vi "2014FullVi.vi"() -> ()   [LabVIEW 2014]
doc: "Use this template to build a standard state machine design pattern. Each state executes code and determines which state to transition to. Contrast this design pattern with the User Interface Event Handler pattern, in which code executes in response to user actions. Contrast this design pattern also with the Queued Message Handler pattern, in which each message handling code can queue zero or more new messages.\nNote: This template does not contain the most recent programming guidelines recommended by National Instruments. For a complete, project-based implementation of the Standard State Machine pattern, use the Create Project dialog box instead of this template."
uses:
  <vilib>/Math Plots/3D Math Plots/3D Bar/3D Bar Datatype/3D Bar Datatype.lvclass
  <vilib>/Math Plots/3D Math Plots/3D Bar/3D Bar Datatype/Public/Plot Helper (Vector).vi
  <vilib>/express/express arith-compare/Formula/XNode/ExpressFormulaBlockNode.xnode
  <vilib>/University of Leeds/Kinesthesia Toolkit for Microsoft Kinect/_Polymorphic Configure/Event-Depth, Skeleton and Video.vi
  <vilib>/University of Leeds/Kinesthesia Toolkit for Microsoft Kinect/_Polymorphic Read/Read-Depth, Skeleton and Video.vi
  <vilib>/Math Plots/3D Math Plots/3D Bar/3D Bar XCtrl/3D Bar.xctl
  Control 1.ctl
panel:
  in  "Which Joint? (2)":T1(ring)
  out "Joint Coordinates (2)":dbl[](array[numeric])
  out "Joint Coordinates (1)":dbl[](array[numeric])
  in  "Which Joint? (1)":T1(ring)
  out "Base DD":dbl[](array[numeric])
  out "Total DD":dbl[](array[numeric])
  in  "1/2 Twist":dbl[](array[numeric])
  in  "360 Somersault":T2
  in  "1/4 Rotation":dbl[](array[numeric])
  in  "Position":string[](array[combo])
  in  "Skill":string[](array[combo])
  in  "FIG Shorthand":string[](array[string])
  out "Average Jump Time":dbl format="%#.3g"
  out "Standard \nDeviation":dbl format="%#.4g"
  out "Tramp contact":bool
  out "?":refnum<class "3D Plot Datatype.lvclass">[](xcontrol)
  out "Total Air Time":dbl format="%#.3g"
  out "Number of Total Jumps":i32
  out "Number of Official Jumps":i32
  in  "Start Official Jumps":bool
  out "Final Jump Times":dbl[](array[numeric])
  out "Trampoline Time":dbl[](array[numeric])
  out "Air Time":dbl[](array[numeric])
  in  "Stop":bool
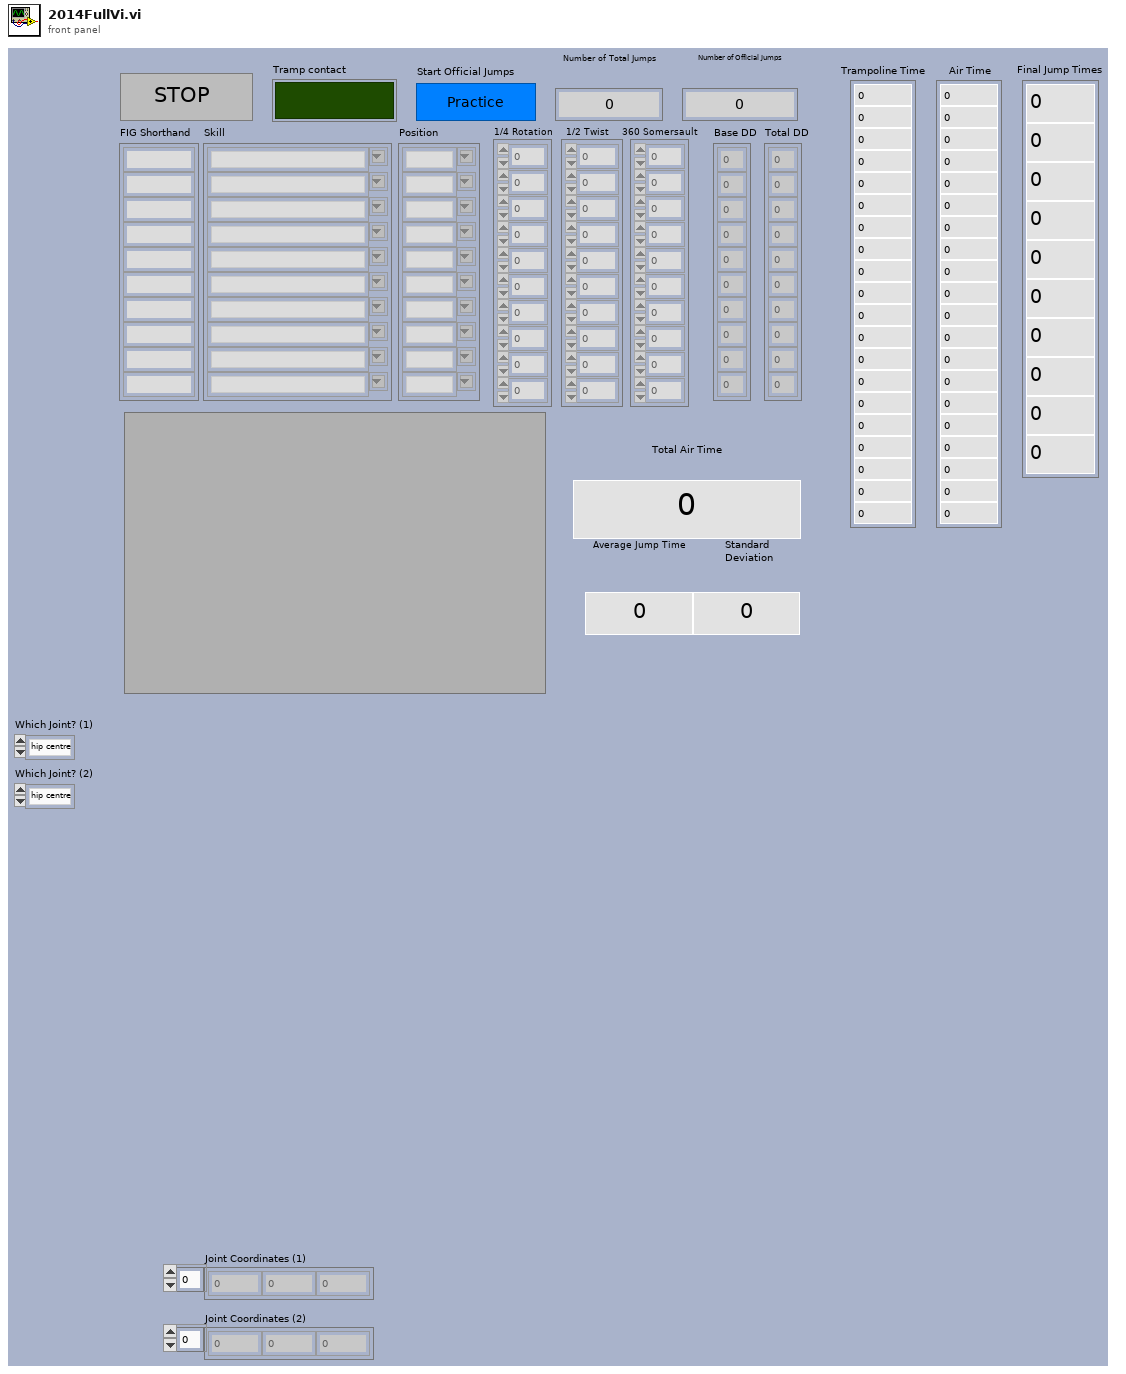
[diagram p1: front panel]
types:
  T1 = enum16{"hip centre", "spine", "shoulder centre", "head", "shoulder left", "elbow left", "wrist left", "hand left", "shoulder right", "elbow right", "wrist right", "hand right", "hip left", "knee left", "ankle left", "foot left", "hip right", "knee right", "ankle right", "foot right"}
  T2 = typedef "Control 1.ctl" = dbl[]
  T3 = cluster{"Start Time":dbl, "Air Time Array ":dbl[], "Tramp Time Array":dbl[], "Number of Jumps  ":i32, "Final Time Array":dbl[], "Number of Final Jumps":i32, "Tramp switch":bool}
  T4 = enum16{"Initialize", "acquire", "analyze", "display", "Stop"}
  T5 = cluster{cluster{"reference out":refnum<k24>, "KinectSensors":refnum<k24>}, "get_Item":refnum<k24>}
  T6 = cluster{"reference out":refnum<k24>, "KinectSensors":refnum<k24>, "SkeletonStream":refnum<k24>, "DepthStream":refnum<k24>, "ColorStream":refnum<k24>, refnum<k24>[], "get_Item":refnum<k24>}
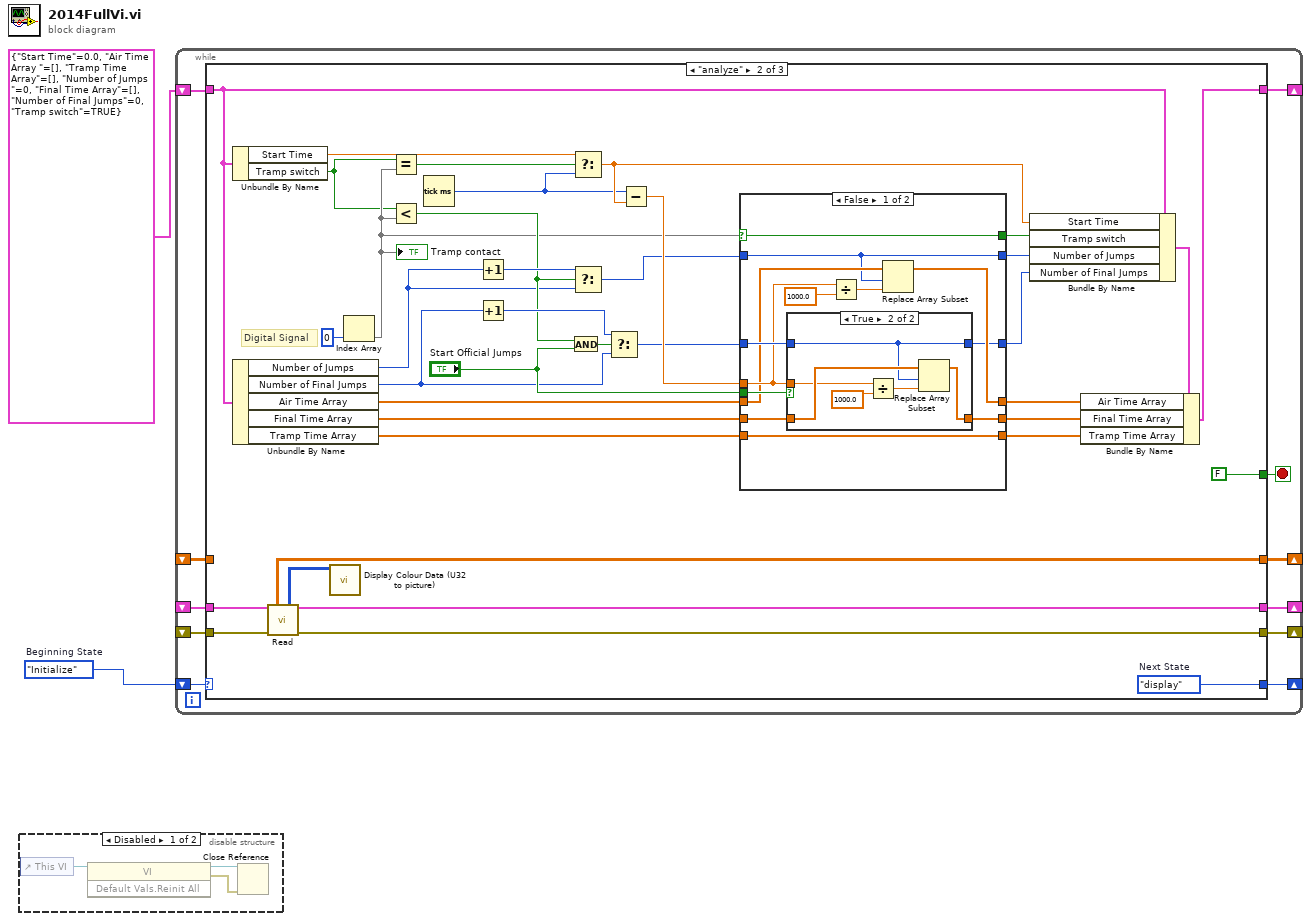
[diagram p0: block diagram]
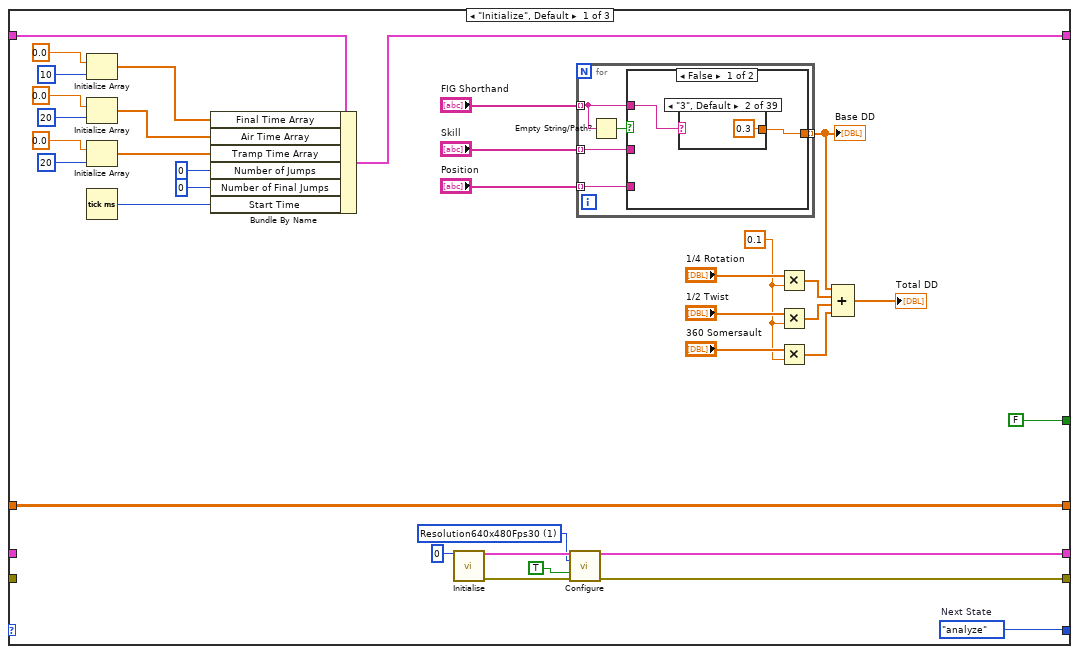
[diagram p3: hidden frame]
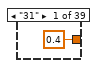
[diagram p4: hidden frame]
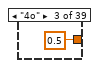
[diagram p5: hidden frame]
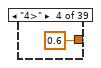
[diagram p6: hidden frame]
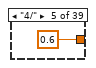
[diagram p7: hidden frame]
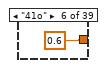
[diagram p8: hidden frame]
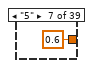
[diagram p9: hidden frame]
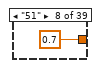
[diagram p10: hidden frame]
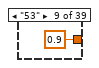
[diagram p11: hidden frame]
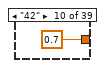
[diagram p12: hidden frame]
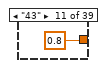
[diagram p13: hidden frame]
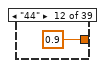
[diagram p14: hidden frame]
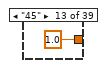
[diagram p15: hidden frame]
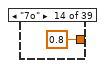
[diagram p16: hidden frame]
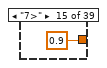
[diagram p17: hidden frame]
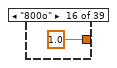
[diagram p18: hidden frame]
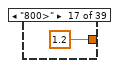
[diagram p19: hidden frame]
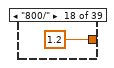
[diagram p20: hidden frame]
diagram:
  w2 = T4."Initialize"  # Beginning State
  n1 = disable-structure shown="Disabled" {
    frame Disabled {
      n2 = control-ref of="This VI"() -> (w5:refnum<vi>)
      n3 = invoke class="VI" method="Default Vals.Reinit All"(reference=w5) -> (reference out=w4:refnum<vi>, error out=w3:errorcluster)  [unwired: 2 in, 1 out]
      n4 = Close Reference(reference=w4, error in (no error)=w3) -> ()  [unwired: 1 out]
    }
    frame Enabled {
    }
  }
  n5 = while {
    shift-right: [w13] -> _
    shift-left: w2 -> [w16]
    shift-right: [w14] -> _
    shift-left: T3 {"Start Time"=0.0, "Air Time Array "=[], "Tramp Time Array"=[], "Number of Jumps  "=0, "Final Time Array"=[], "Number of Final Jumps"=0, "Tramp switch"=TRUE} -> [w15]
    shift-right: [w11] -> _
    shift-left: _ -> [w9]
    shift-right: [w10] -> _
    shift-left: _ -> [w8]
    shift-right: [w7] -> _
    shift-left: _ -> [w6]
    stop <- w12 stop-if-true
    n6 = case shown="\"analyze\"" w16 {
      tunnel: [w52 w224 w284] -> w13
      tunnel: w15 -> [w51 w209 w281]
      tunnel: [w43 w201 w281] -> w14
      tunnel: [FALSE FALSE w282] -> w12
      tunnel: [w19 w188 w256] -> w11
      tunnel: [w18 w189 w258] -> w10
      tunnel: w9 -> [_ w191 w256]
      tunnel: w8 -> [_ w190 w259]
      tunnel: [w17 w187 w257] -> w7
      tunnel: w6 -> [w17 _ w257]
      frame "Initialize", Default {
        w21 = 1 items=["Undefined", "Resolution640x480Fps30", "Resolution320x240Fps30", "Resolution80x60Fps30"] ("Depth Stream Format")
        w28 = 0.1
        w52 = T4."analyze"  # Next State
        n7 = Initialize Array(0.0 ("element"), 10 ("dimension size")) -> (w40:dbl[])
        n8 = Initialize Array(0.0 ("element"), 20 ("dimension size")) -> (w47:dbl[])
        n9 = Initialize Array(0.0 ("element"), 20 ("dimension size")) -> (w44:dbl[])
        n10 = Tick Count (ms)() -> (millisecond timer value=w37:u32)
        n11 = Bundle By Name(cluster=w51, "Final Time Array"=w40, "Air Time Array"=w47, "Tramp Time Array"=w44, "Number of Jumps"=0 ("Tramp release"), "Number of Final Jumps"=0, "Start Time"=w37) -> (w43:T3)
        n12 = call <vilib>:"Initialise.vi"("Kinect Number"=0) -> ("Kinect References out"=w24:T5, "error out"=w23:errorcluster)  [unwired: 13 in]
        n13 = call-poly <vilib>:"Configure.vi"("Kinect References in"=w24, "Depth Stream Format"=w21, "Skeleton Smoothing"=TRUE, "error in"=w23) -> ("Kinect References out"=w19:T6, "error out"=w18:errorcluster)  [unwired: 10 in]
        n14 = for {
          tunnel: "FIG Shorthand" -> [w55] mode=indexing
          tunnel: [w57] -> w29 mode=indexing
          tunnel: "Skill" -> [w54] mode=indexing
          tunnel: "Position" -> [w53] mode=indexing
          n15 = Empty String/Path?(string/path=w55) -> (empty?=w56:bool)
          n16 = case shown="False" w56 {
            tunnel: w55 -> [w59 _]
            tunnel: [w58 w99] -> w57
            tunnel: w54 -> [_ w101]
            tunnel: w53 -> [_ w100]
            frame False {
              n17 = case shown="\"3\", Default" w59 {
                tunnel: [0.4 0.3 0.5 0.6 0.6 0.6 0.6 0.7 0.9 0.7 0.8 0.9 1.0 0.8 0.9 1.0 1.2 1.2 1.1 1.1 1.3 1.3 1.5 1.3 1.5 1.7 2.0 0.6 0.7 0.8 1.1 1.2 1.4 1.4 1.6 1.2 1.4 1.4 1.6] -> w58
                frame "31" {
                }
                frame "3", Default {
                }
                frame "4o" {
                }
                frame "4>" {
                }
                frame "4/" {
                }
                frame "41o" {
                }
                frame "5" {
                }
                frame "51" {
                }
                frame "53" {
                }
                frame "42" {
                }
                frame "43" {
                }
                frame "44" {
                }
                frame "45" {
                }
                frame "7o" {
                }
                frame "7>" {
                }
                frame "800o" {
                }
                frame "800>" {
                }
                frame "800/" {
                }
                frame "810o" {
                }
                frame "801o" {
                }
                frame "801>" {
                }
                frame "821o" {
                }
                frame "821/" {
                }
                frame "803o" {
                }
                frame "803>" {
                }
                frame "12001o" {
                }
                frame "12001>" {
                }
                frame "5o" {
                }
                frame "5>" {
                }
                frame "52" {
                }
                frame "46" {
                }
                frame "802o" {
                }
                frame "802/" {
                }
                frame "822o" {
                }
                frame "822/" {
                }
                frame "811o" {
                }
                frame "811>" {
                }
                frame "813o" {
                }
                frame "813>" {
                }
              }
            }
            frame True {
              n18 = case shown="\"Full Out\"" w101 {
                tunnel: w100 -> [_ _ w104 w109 _ _ _ _ _ _ _ w121 w125 _ w131 w135 w139 w143 _ w149 w154 _ _ _ _ w163 w166 w171 w175 w179 w184]
                tunnel: [0.3 0.4 w105 w110 0.6 0.7 0.9 0.7 0.8 0.9 1.0 w122 w126 1.1 w132 w136 w140 w144 0.3 w148 w153 0.7 0.8 0.9 1.1 w162 w167 w172 w176 w180 w183] -> w99
                frame "3/4 Front", Default {
                }
                frame "Arabian 3/4 Front" {
                }
                frame "Front" {
                  n19 = case shown="\"Straight\"" w104 {
                    tunnel: [0.6 0.6 0.5] -> w105
                    frame "Straight" {
                    }
                    frame "Pike" {
                    }
                    frame "Tuck", Default {
                    }
                  }
                }
                frame "Barani" {
                  n20 = case shown="\"Straight\"" w109 {
                    tunnel: [0.6 0.6 0.6] -> w110
                    frame "Straight" {
                    }
                    frame "Pike" {
                    }
                    frame "Tuck", Default {
                    }
                  }
                }
                frame "Ballout" {
                }
                frame "Barani Ballout" {
                }
                frame "Rudy Ballout" {
                }
                frame "Front Full" {
                }
                frame "Rudi" {
                }
                frame "Front Double Full" {
                }
                frame "Randi" {
                }
                frame "1 3/4 Front" {
                  n21 = case shown="\"Tuck\", Default" w121 {
                    tunnel: [0.9 0.8] -> w122
                    frame "Pike" {
                    }
                    frame "Tuck", Default {
                    }
                  }
                }
                frame "Double Front" {
                  n22 = case shown="\"Pike\"" w125 {
                    tunnel: [1.2 1.2 1.0] -> w126
                    frame "Straight" {
                    }
                    frame "Pike" {
                    }
                    frame "Tuck", Default {
                    }
                  }
                }
                frame "Half In Back Out" {
                }
                frame "Half Out" {
                  n23 = case shown="\"Tuck\", Default" w131 {
                    tunnel: [1.3 1.1] -> w132
                    frame "Pike" {
                    }
                    frame "Tuck", Default {
                    }
                  }
                }
                frame "Full Barani" {
                  n24 = case shown="\"Tuck\", Default" w135 {
                    tunnel: [1.5 1.1] -> w136
                    frame "Straight" {
                    }
                    frame "Tuck", Default {
                    }
                  }
                }
                frame "Rudi Out" {
                  n25 = case shown="\"Tuck\", Default" w139 {
                    tunnel: [1.5 1.3] -> w140
                    frame "Pike" {
                    }
                    frame "Tuck", Default {
                    }
                  }
                }
                frame "Triffus" {
                  n26 = case shown="\"Tuck\", Default" w143 {
                    tunnel: [2.0 1.7] -> w144
                    frame "Pike" {
                    }
                    frame "Tuck", Default {
                    }
                  }
                }
                frame "3/4 Back" {
                }
                frame "Back" {
                  n27 = case shown="\"Straight\"" w149 {
                    tunnel: [0.6 0.6 0.5] -> w148
                    frame "Pike" {
                    }
                    frame "Straight" {
                    }
                    frame "Tuck", Default {
                    }
                  }
                }
                frame "Cody" {
                  n28 = case shown="\"Straight\"" w154 {
                    tunnel: [0.7 0.8 0.6] -> w153
                    frame "Pike" {
                    }
                    frame "Straight" {
                    }
                    frame "Tuck", Default {
                    }
                  }
                }
                frame "Back Full" {
                }
                frame "Back 1 1/2 Full" {
                }
                frame "Back Double Full" {
                }
                frame "Back Triple Full" {
                }
                frame "1 3/4 Back" {
                  n29 = case shown="\"Tuck\", Default" w163 {
                    tunnel: [0.9 0.8] -> w162
                    frame "Pike" {
                    }
                    frame "Tuck", Default {
                    }
                  }
                }
                frame "Double Back" {
                  n30 = case shown="\"Tuck\", Default" w166 {
                    tunnel: [1.2 1.2 1.0] -> w167
                    frame "Straight" {
                    }
                    frame "Pike" {
                    }
                    frame "Tuck", Default {
                    }
                  }
                }
                frame "Full Out" {
                  n31 = case shown="\"Tuck\", Default" w171 {
                    tunnel: [1.4 1.2] -> w172
                    frame "Straight" {
                    }
                    frame "Tuck", Default {
                    }
                  }
                }
                frame "Full Full" {
                  n32 = case shown="\"Tuck\", Default" w175 {
                    tunnel: [1.6 1.4] -> w176
                    frame "Straight" {
                    }
                    frame "Tuck", Default {
                    }
                  }
                }
                frame "Half Half" {
                  n33 = case shown="\"Tuck\", Default" w179 {
                    tunnel: [1.4 1.2] -> w180
                    frame "Pike" {
                    }
                    frame "Tuck", Default {
                    }
                  }
                }
                frame "Half Rudi" {
                  n34 = case shown="\"Tuck\", Default" w184 {
                    tunnel: [1.6 1.4] -> w183
                    frame "Pike" {
                    }
                    frame "Tuck", Default {
                    }
                  }
                }
              }
            }
          }
        }
        "Base DD" <- w29
        n35 = Multiply(x="1/4 Rotation", y=w28) -> (x*y=w33:dbl[])
        n36 = Multiply(x="1/2 Twist", y=w28) -> (x*y=w32:dbl[])
        n37 = Multiply(x="360 Somersault", y=w28) -> (x*y=w31:T2)
        n38 = Compound Arithmetic op=ADD(w29, w33, w32, w31) -> (→"Total DD":T2)
      }
      frame "analyze" {
        w224 = T4."display"  # Next State
        # "Digital Signal"
        n39 = Unbundle By Name(w209) -> ("Start Time"=w199:dbl, "Tramp switch"=w193:bool)
        n40 = Unbundle By Name(w209) -> ("Number of Jumps"=w197:i32, "Number of Final Jumps"=w198:i32, "Air Time Array"=w214:dbl[], "Final Time Array"=w213:dbl[], "Tramp Time Array"=w207:dbl[])
        n41 = call-poly <vilib>:"Read.vi"("Kinect References in"=w191, "error in (no error)"=w190) -> ("Primary Skeleton Array"=w187:dbl[][], "Colour output array (U24, RGB)"=w192:u32[][], "Kinect References out"=w188:T6, "error out"=w189:errorcluster)  [unwired: 8 in, 2 out]
        n42 = call <vilib>:"Display Colour Data (U32 to picture).vi"("Colour output array (U24, RGB)"=w192) -> ()  [unwired: 10 in, 1 out]
        n43 = Index Array(index=0) -> (array=w196:bool[], element=w194)
        "Tramp contact" <- w194
        n44 = Equal?(x=w193, y=w194) -> (x = y?=w221:bool)
        n45 = Less?(x=w193, y=w194) -> (x < y?=w211:bool)
        n46 = Tick Count (ms)() -> (millisecond timer value=w200:u32)
        n47 = Increment(x=w197) -> (x+1=w222:i32)
        n48 = Increment(x=w198) -> (x+1=w218:i32)
        n49 = And(x=w211, y="Start Official Jumps") -> (x .and. y?=w216:bool)
        n50 = Select(t=w199, s=w221, f=w200) -> (s? t:f=w212:dbl)
        n51 = Select(t=w222, s=w211, f=w197) -> (s? t:f=w215:i32)
        n52 = Select(t=w218, s=w216, f=w198) -> (s? t:f=w217:i32)
        n53 = Subtract(x=w200, y=w212) -> (x-y=w220:dbl)
        n54 = case shown="False" w194 {
          selector: w194 -> [w225 w248]
          tunnel: [w226 w251] -> w203
          tunnel: [w237 w246] -> w205
          tunnel: w213 -> [w228 w247]
          tunnel: w215 -> [w227 w250]
          tunnel: w220 -> [w230 w253]
          tunnel: w214 -> [w229 w246]
          tunnel: [w236 w247] -> w206
          tunnel: w217 -> [w235 w255]
          tunnel: [w234 w255] -> w219
          tunnel: "Start Official Jumps" -> [w233 _]
          tunnel: [w227 w250] -> w208
          tunnel: w207 -> [w226 w249]
          tunnel: [w225 w248] -> w204
          frame False {
            n55 = case shown="True" w233 {
              tunnel: w230 -> [_ w241]
              tunnel: [w239 w244] -> w236
              tunnel: w228 -> [w239 w245]
              tunnel: w235 -> [w238 w240]
              tunnel: [w238 w240] -> w234
              frame False {
              }
              frame True {
                n56 = Divide(x=w241, y=1000.0) -> (x/y=w242:dbl)
                n57 = Replace Array Subset(array=w245, new element=w242, index=w240) -> (w244:dbl[])
              }
            }
            n58 = Divide(x=w230, y=1000.0) -> (x/y=w231:dbl)
            n59 = Replace Array Subset(array=w229, new element=w231, index=w227) -> (w237:dbl[])
          }
          frame True {
            # "This true case is tramp time array"
            n60 = Divide(x=w253, y=1000.0) -> (x/y=w252:dbl)
            n61 = Replace Array Subset(array=w249, new element=w252, index=w250) -> (w251:dbl[])
          }
        }
        n62 = Bundle By Name(cluster=w209, "Start Time"=w212, "Tramp switch"=w204, "Number of Jumps"=w208, "Number of Final Jumps"=w219) -> (w202:T3)
        n63 = Bundle By Name(cluster=w202, "Air Time Array"=w205, "Final Time Array"=w206, "Tramp Time Array"=w203) -> (w201:T3)
      }
      frame "display" {
        w284 = T4."analyze"  # Next State
        n64 = Unbundle By Name(w281) -> ("Air Time Array"=→"Air Time":dbl[], "Tramp Time Array"=→"Trampoline Time":dbl[], "Final Time Array"=w272:dbl[])
        "Final Jump Times" <- w272
        n65 = call <vilib>:"Joint Coordinates.vi"("error in (no error)"=w259, "Joint 1"="Which Joint? (1)", "Array of Joint Positions"=w257) -> ("error out"=w260:errorcluster, "Joint Coordinates"=→"Joint Coordinates (1)":dbl[])  [unwired: 7 in]
        n66 = Add Array Elements(numeric array=w272) -> (sum=w271:dbl)
        "Total Air Time" <- w271
        n67 = Divide(x=w271, y=10.0) -> (x/y=w265:dbl)
        "Average Jump Time" <- w265
        n68 = call-poly <vilib>:"Plot Helper.vi"("z vector"=w272, "y vector"=sgl[] [1.0, 2.0, 3.0, 4.0, 5.0, 6.0, 7.0, 8.0, 9.0, 10.0]) -> ("3D Plot lvclass Array out"=→"?":refnum<class "3D Plot Datatype.lvclass">[])  [unwired: 1 in, 8 out]
        n69 = Unbundle By Name(w281) -> ("Number of Jumps"=→"Number of Total Jumps":i32, "Number of Final Jumps"=w279:i32)
        "Number of Official Jumps" <- w279
        n70 = call <vilib>:"Joint Coordinates.vi"("error in (no error)"=w260, "Joint 1"="Which Joint? (2)", "Array of Joint Positions"=w257) -> ("error out"=w258:errorcluster, "Joint Coordinates"=→"Joint Coordinates (2)":dbl[])  [unwired: 7 in]
        n71 = for {
          N: 10 -> [_]
          tunnel: w272 -> [w286] mode=indexing
          tunnel: w265 -> [w287]
          tunnel: [w285] -> w269 mode=indexing
          n72 = xnode "Formula"("Jump Time"=w286, "Average"=w287) -> ("Result"=w285:dbl)  [unwired: 1 in, 1 out]
        }
        n73 = Add Array Elements(numeric array=w269) -> (sum=w267:dbl)
        n74 = Square Root(x=w267) -> (sqrt(x)=→"Standard \nDeviation":dbl)
        n75 = Greater Or Equal?(x=w279, y=10) -> (x >= y?=w274:bool)
        n76 = Or(x=w274, y="Stop") -> (x .or. y?=w282:bool)
      }
    }
  }
